vi "Read Stream.vi"(6 "Timout (s)":i32, 8 "error in (no error)":errorcluster, 9 "Connection Name":string, 10 "Expected Response":string, 11 "Output ref":refnum<vi>) -> (0 "error out":errorcluster)   [LabVIEW 2015, in "LabSSH.lvlib"]
doc: "<License>This software is distributed under the BSD 3-Clause License. For the full license please see license.txt or visit www.labvolution.com/license</License>"
uses:
  LabSSH.lvlib
  FGV State..enum.ctl
  C:/Working Folder/ssh.git/LabSSH Library/References/Renci.SshNet.dll
  References/Renci.SshNet.dll
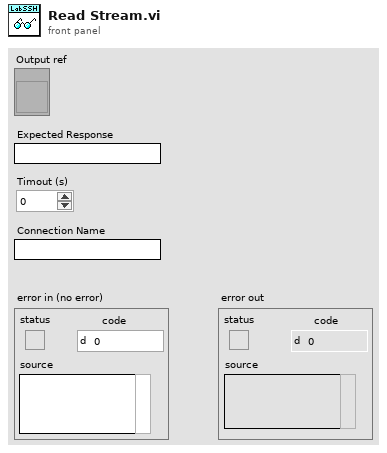
[diagram p1: front panel]
types:
  T1 = typedef "LabSSH.lvlib/FGV State..enum.ctl" = enum16{"GET", "SET"}
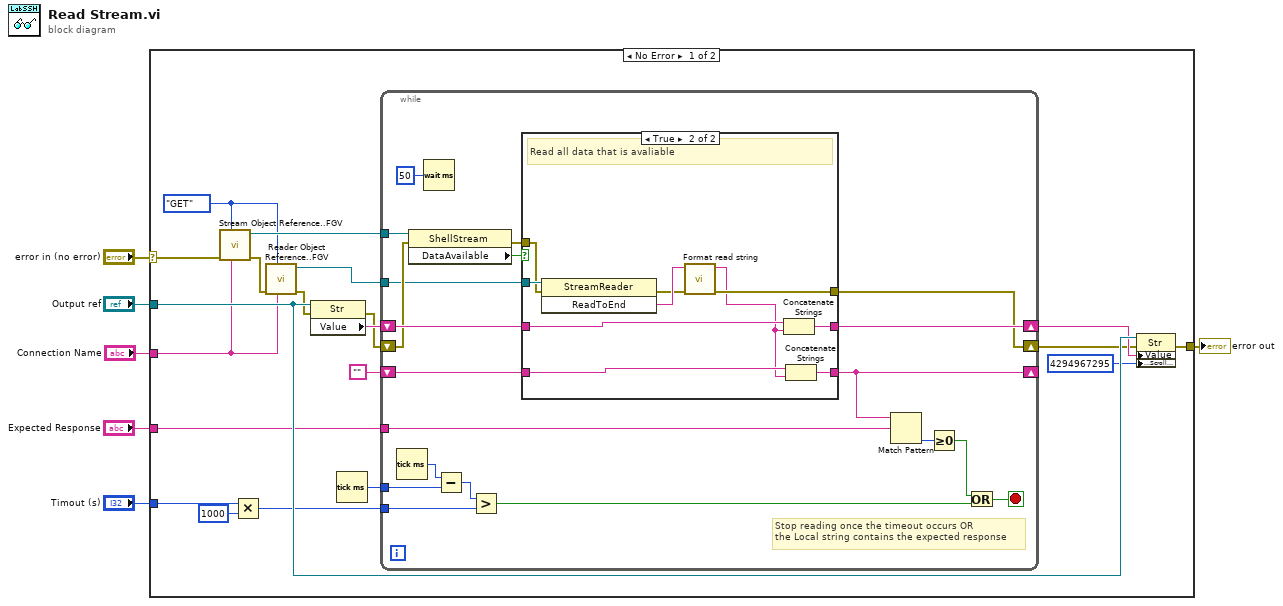
[diagram p0: block diagram]
diagram:
  n1 = case shown="No Error" "error in (no error)" {
    selector: "error in (no error)" -> [w15 w60]
    tunnel: "Timout (s)" -> [w13 _]
    tunnel: "Output ref" -> [w25 _]
    tunnel: [w20 w60] -> w4
    tunnel: "Expected Response" -> [w9 _]
    tunnel: "Connection Name" -> [w7 _]
    frame No Error {
      w16 = FGV_State..enum."GET" ("FGV State")
      n2 = call "Stream Object Reference..FGV.vi"("Connection Name"=w7, "FGV State (GET)"=w16, "error in (no error)"=w15) -> ("error out"=w18:errorcluster, "Stream ref out"=w23:refnum<k24>)  [unwired: 7 in]
      n3 = Multiply(x=w13, y=1000) -> (x*y=w11:i32)
      n4 = call "Reader Object Reference..FGV.vi"("Connection Name"=w7, "FGV State (GET)"=w16, "error in (no error)"=w18) -> ("error out"=w17:errorcluster, "Reader ref out"=w22:refnum<k24>)  [unwired: 7 in]
      n5 = property class="Str"(reference=w25, error in=w17) -> (error out=w19:errorcluster, "Value"=w26:string)  [unwired: 1 out]
      n6 = Tick Count (ms)() -> (millisecond timer value=w14:u32)
      n7 = while {
        tunnel: w23 -> [w45]
        tunnel: w22 -> [w41]
        shift-right: [w39] -> w24
        shift-left: w26 -> [w43]
        shift-right: [w38] -> w21
        shift-left: w19 -> [w42]
        tunnel: w14 -> [w37]
        tunnel: w11 -> [w34]
        shift-right: [w30] -> _
        shift-left: "" -> [w32]
        tunnel: w9 -> [w29]
        stop <- w31 stop-if-true
        # "Stop reading once the timeout occurs OR\nthe Local string contains the expected response"
        n8 = Tick Count (ms)() -> (millisecond timer value=w36:u32)
        n9 = property class="ShellStream"(reference=w45, error in=w42) -> (error out=w40:errorcluster, "DataAvailable"=w44:bool)  [unwired: 1 out]
        n10 = Wait (ms)(milliseconds to wait=u32 50) -> ()  [unwired: 1 out]
        n11 = Subtract(x=w36, y=w37) -> (x-y=w35:u32)
        n12 = Greater?(x=w35, y=w34) -> (0:w33:bool)
        n13 = case shown="True" w44 {
          tunnel: w43 -> [w49 w57]
          tunnel: w41 -> [_ w59]
          tunnel: w40 -> [w48 w58]
          tunnel: [w49 w56] -> w39
          tunnel: [w48 w51] -> w38
          tunnel: w32 -> [w47 w55]
          tunnel: [w47 w54] -> w30
          frame False {
          }
          frame True {
            # "Read all data that is avaliable"
            n14 = invoke class="StreamReader" method="ReadToEnd"(reference=w59, error in=w58) -> (error out=w52:errorcluster, "ReadToEnd"=w53:string)  [unwired: 1 in, 1 out]
            n15 = call "Format read string.vi"("error in (no error)"=w52, "Input String"=w53) -> ("error out"=w51:errorcluster, "Formatted Output String"=w50:string)  [unwired: 8 in]
            n16 = Concatenate Strings(w57, w50) -> (w56:string)
            n17 = Concatenate Strings(w55, w50) -> (w54:string)
          }
        }
        n18 = Match Pattern(string=w30, regular expression=w29) -> (offset past match=w28:i32)  [unwired: 1 in, 3 out]
        n19 = Greater Or Equal To 0?(x=w28) -> (x >= 0?=w27:bool)
        n20 = Or(x=w27, y=w33) -> (x .or. y?=w31:bool)
      }
      n21 = property class="Str"(reference=w25, error in=w21, "Value"=w24, "Text.Scroll Position"=u32 4294967295) -> (error out=w20:errorcluster)  [unwired: 1 out]
    }
    frame Error {
    }
  }
  "error out" <- w4
